vi "Fingerprint.vi"(8 "Error In":errorcluster, 10 "Type":T1=2 items=["MD5"=1, "SHA1"=2], 11 "Session In":refnum<class "Session.lvclass">) -> (0 "Error Out":errorcluster, 2 "Fingerprint":u8[](array[numeric]), 3 "Sesssion Out":refnum<class "Session.lvclass">)   [LabVIEW 2018, in "Toolkit.lvlib" / "Session.lvclass"]
doc: "Gets a hash of the remote SSH server's host key. This is an unique identifier for the remote SSH server, typically referred to as a \"fingerprint\". The server's host key hash can be used to ensure the remote SSH server is valid, recognized, and geninue. If the fingerprint does not match an existing, known remote SSH server's host key hash, then do NOT proceed with authentication."
uses:
  Session.lvclass
  Typedefs/Host Key Hash Types.ctl
  Session.lvclass/Session.ctl
  SSH/SSH.lvclass/SSH.ctl
  Toolkit.lvlib
  SSH/SSH.lvclass
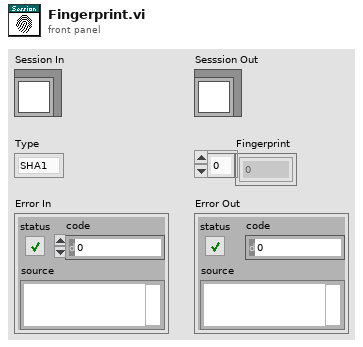
[diagram p1: front panel]
types:
  T1 = typedef "Toolkit.lvlib/Session.lvclass/Host Key Hash Types.ctl" = i32
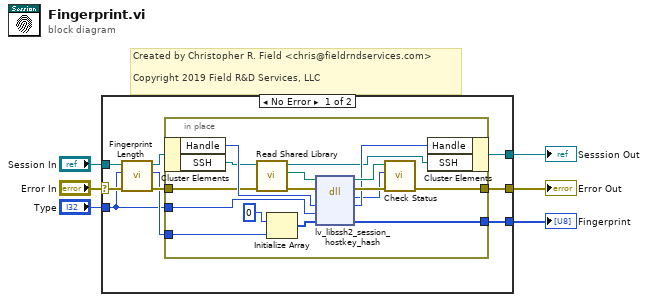
[diagram p0: block diagram]
diagram:
  # "Created by Christopher R. Field <chris@fieldrndservices.com>\n\nCopyright 2019 Field R&D Services, LLC"
  n1 = case shown="No Error" "Error In" {
    selector: "Error In" -> [w10 w33]
    tunnel: [w14 w33] -> w5
    tunnel: "Session In" -> [w12 w32]
    tunnel: [w15 w32] -> w3
    tunnel: [w13 _] -> w2
    tunnel: "Type" -> [w7 _]
    frame No Error {
      n2 = call "Fingerprint Length.vi"("Error In"=w10, "Type"=w7, "Session In"=w12) -> ("Error Out"=w9:errorcluster, "Length"=w8:i32, "Sesssion Out"=w11:refnum<class "Session.lvclass">)  [unwired: 6 in]
      n3 = in-place {
        in-place-border: [w29] -> w14
        in-place-border: [w23] -> w13
        in-place-border: w9 -> [w22]
        in-place-border: w8 -> [w21]
        in-place-border: w7 -> [w16]
        n4 = in-place-cluster #1(w11) -> ("Handle"=w28:u64, "SSH"=w19:refnum<class "SSH.lvclass">)
        n5 = call "Read Shared Library.vi"("Error In"=w22, "SSH In"=w19) -> ("Error Out"=w20:errorcluster, "lv-libssh2 Shared Library"=w18:path, "SSH Out"=w17:refnum<class "SSH.lvclass">)  [unwired: 7 in]
        n6 = Initialize Array(u8 0, w21) -> (w25:u8[])
        n7 = dll-call lib="D:/Users/cfield/Code/Field R&D Services/SSH/LabSSH2/LabVIEW/trunk/src/Toolkit/Support/lv-libssh2.*" fn="lv_libssh2_session_hostkey_hash"(path in=w18, error in=w20, "session"=w28, "type"=w16, "buffer"=w25) -> (path out=w31:path, error out=w30:errorcluster, "result"=w24:i32, "session"=w27:u64, "buffer"=w23:u8[])  [unwired: 2 in]
        n8 = call "Check Status.vi"("Error In"=w30, "Status"=w24, "lv-libssh2 Shared Library In"=w31) -> ("Error Out"=w29:errorcluster)  [unwired: 7 in, 1 out]
        n9 = in-place-cluster #1("Handle"=w27, "SSH"=w17) -> (w15:refnum<class "Session.lvclass">)
      }
    }
    frame Error {
    }
  }
  "Sesssion Out" <- w3
  "Error Out" <- w5
  "Fingerprint" <- w2
